vi "aggiorna banco e progressivo acquisizioni.vi"(9 "banco":string, 10 "progressivo":string, 11 "Dati":string[][](array[string])) -> (3 "Dati out":string[][](array[string]))   [LabVIEW 2019]
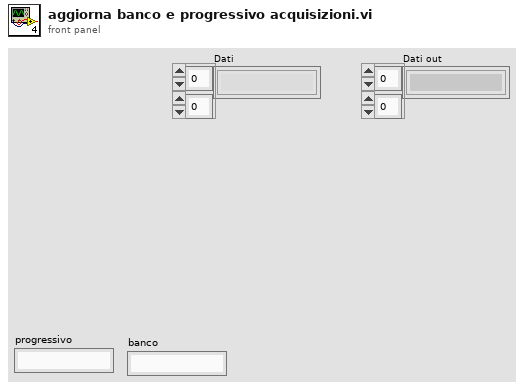
[diagram p1: front panel]
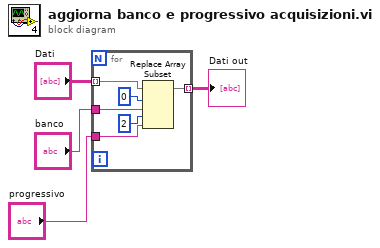
[diagram p0: block diagram]
diagram:
  n1 = for {
    tunnel: "Dati" -> [w10] mode=indexing
    tunnel: "banco" -> [w8]
    tunnel: "progressivo" -> [w6]
    tunnel: [w5] -> w4 mode=indexing
    n2 = Replace Array Subset(array=w10, new element #1=w8, index #1=0 ("disabled index (col)"), new element #2=w6, index #2=2 ("index")) -> (w5:string[])
  }
  "Dati out" <- w4
